vi "Wrapper_closeAllSpectrometers_Mod.vi"(8 "error in (no error)":errorcluster caption="entrée d'erreur (pas d'erreur)", 10 "Wrapper In":u32) -> (0 "error out":errorcluster caption="sortie d'erreur", 2 "Wrapper Out":u32)   [LabVIEW 2024]
uses:
  OmniDriver32.dll
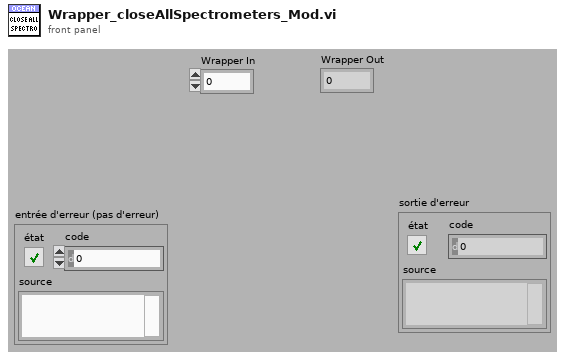
[diagram p1: front panel]
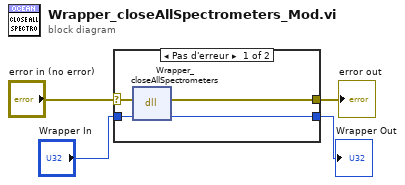
[diagram p0: block diagram]
diagram:
  n1 = case shown="Pas d'erreur" "error in (no error)" {
    selector: "error in (no error)" -> [w6 w10]
    tunnel: "Wrapper In" -> [w8 w9]
    tunnel: [w7 w9] -> w3
    tunnel: [w5 w10] -> w1
    frame No Error {
      n2 = dll-call lib="OmniDriver32.dll" fn="Wrapper_closeAllSpectrometers" label="Wrapper.closeAllSpectrometers"(error in=w6, "Wrapper"=w8) -> (error out=w5:errorcluster, "Wrapper"=w7:u32)  [unwired: 2 in, 2 out]
    }
    frame Error {
    }
  }
  "Wrapper Out" <- w3
  "error out" <- w1
